vi "set console output.vi"(10 "console_output":string) -> ()   [LabVIEW 2019, in "libSimulationControl.lvlib"]
uses:
  libSimulationControl.lvlib
panel:
  out "error out":errorcluster
  in  "error in (no error)":errorcluster
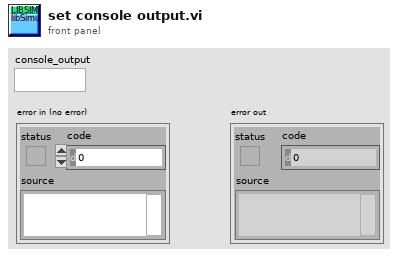
[diagram p1: front panel]
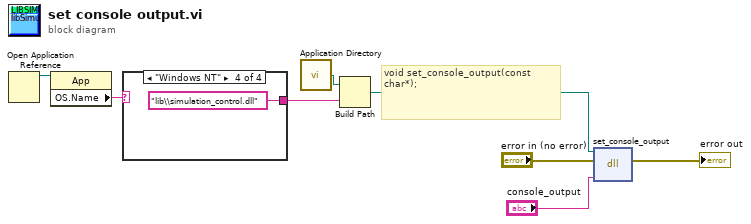
[diagram p0: block diagram]
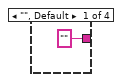
[diagram p2: hidden frame]
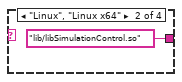
[diagram p3: hidden frame]
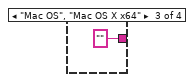
[diagram p4: hidden frame]
diagram:
  # "void set_console_output(const char*);"
  n1 = Open Application Reference() -> (3:w7:refnum<vi>)  [unwired: 4 in, 1 out]
  n2 = property class="App"(reference=w7) -> ("OS.Name"=w6:string)  [unwired: 1 in, 2 out]
  n3 = case shown="\"Windows NT\"" w6 {
    tunnel: ["" ("return type") "lib/libSimulationControl.so" ("name or relative path") "" ("return type") "lib\\simulation_control.dll" ("name or relative path")] -> w5
    frame "", Default {
    }
    frame "Linux", "Linux x64" {
    }
    frame "Mac OS", "Mac OS X x64" {
    }
    frame "Windows NT" {
    }
  }
  n4 = call <vilib>:"Application Directory.vi"() -> ("Application Directory"=w4:path)
  n5 = Build Path(base path=w4, name or relative path=w5) -> (appended path=w3:path)
  n6 = dll-call lib="home/paul/Schreibtisch/Biogas_plant_setup/LabView/lib/libSimulationControl.so" fn="set_console_output"(path in=w3, error in="error in (no error)", "console_output"="console_output") -> (error out=→"error out":errorcluster)  [unwired: 3 in, 1 out]
